vi "Ej 17 PWM_DAQ.vi"() -> ()   [LabVIEW 2021]
panel:
  in  "Amplitud":dbl=1.7 caption="Offset"
  out "Waveform Graph":dynamicdata(graph)
  in  "stop":bool
  in  "Duty Cycle (%)":dbl=5.0
  in  "Frequency":dbl=50.0
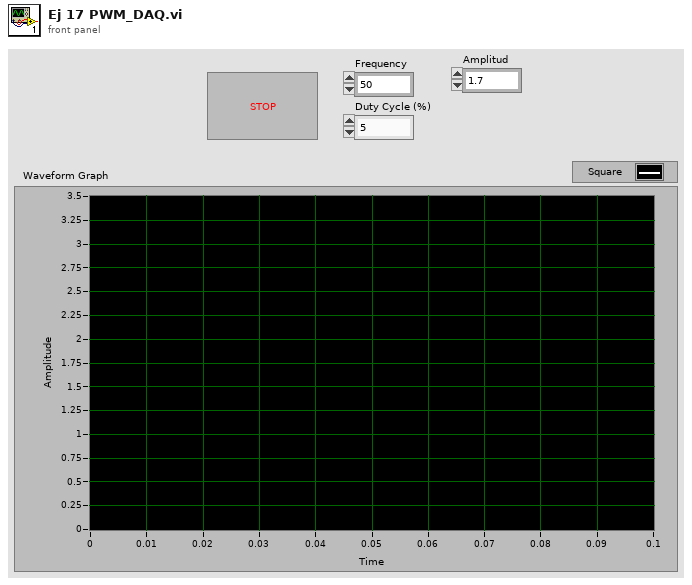
[diagram p1: front panel]
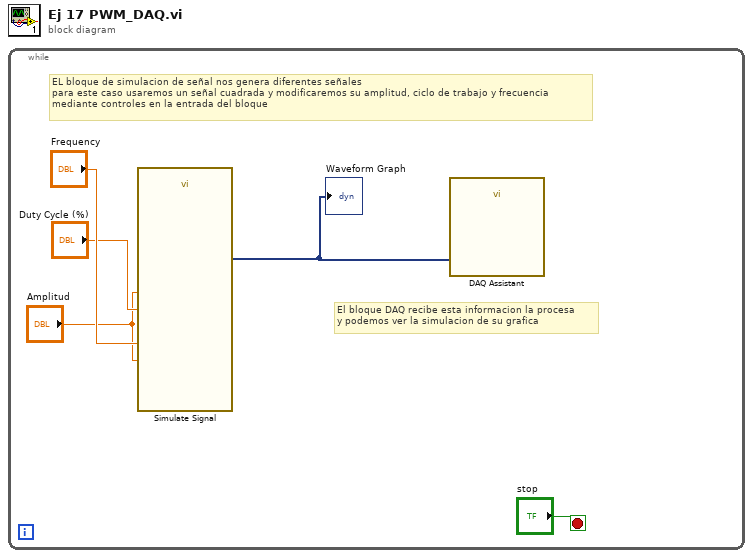
[diagram p0: block diagram]
diagram:
  n1 = while {
    stop <- "stop" stop-if-true
    # "El bloque DAQ recibe esta informacion la procesa\ny podemos ver la simulacion de su grafica"
    # "EL bloque de simulacion de señal nos genera diferentes señales \npara este caso usaremos un señal cuadrada y modificaremos su amplitud, ciclo de trabajo y frecuencia\nmediante controles en la entrada del bloque"
    n2 = call "Simulate Signal"("Offset"="Amplitud", "Duty Cycle (%)"="Duty Cycle (%)", "Frequency"="Frequency", "Amplitude"="Amplitud") -> ("Square"=w2:dynamicdata)  [unwired: 10 in, 1 out]
    "Waveform Graph" <- w2
    n3 = call "DAQ Assistant"("data"=w2) -> ()  [unwired: 17 in, 2 out]
  }
